vi "Set Excel Value.vi"(4 "Excel_Values":string[][](array[string]), 6 "SheetName(\"\")":string, 8 "error in (no error)":errorcluster, 9 "End":cluster{"Column":i32, "Row":i32}={"Column"=8, "Row"=7}, 10 "Start":cluster{"Column":i32, "Row":i32}={"Column"=1, "Row"=1}, 11 "path":path) -> (0 "error out":errorcluster)   [LabVIEW 2015]
uses:
  Private Methods/OpenXL_WorkSheet By Name.vi
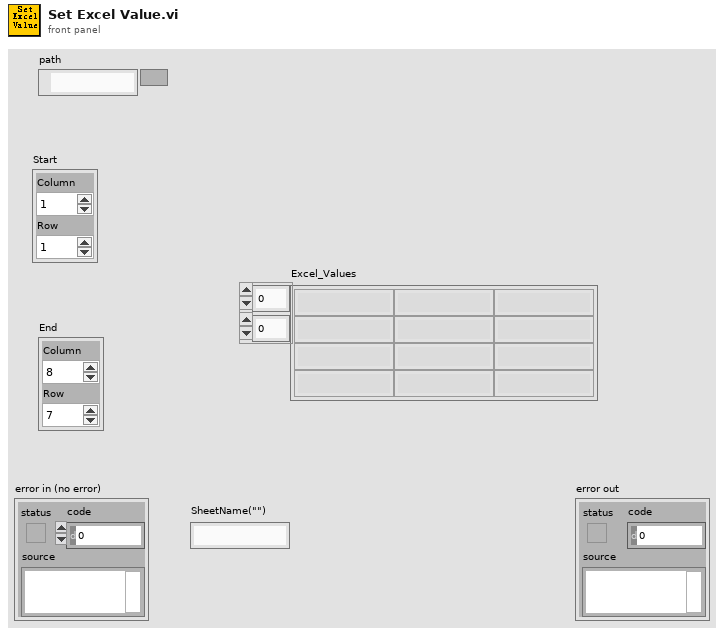
[diagram p1: front panel]
types:
  T1 = cluster{"Excel._Application":refnum<k7>, "Workbooks":refnum<k7>}
  T2 = cluster{"Excel._Application":refnum<k7>, "Workbooks":refnum<k7>, "Open":refnum<k7>}
  T3 = cluster{"Excel._Application":refnum<k7>, "Workbooks":refnum<k7>, "Open":refnum<k7>, "Worksheets":refnum<k7>, "Excel._Worksheet":refnum<k7>}
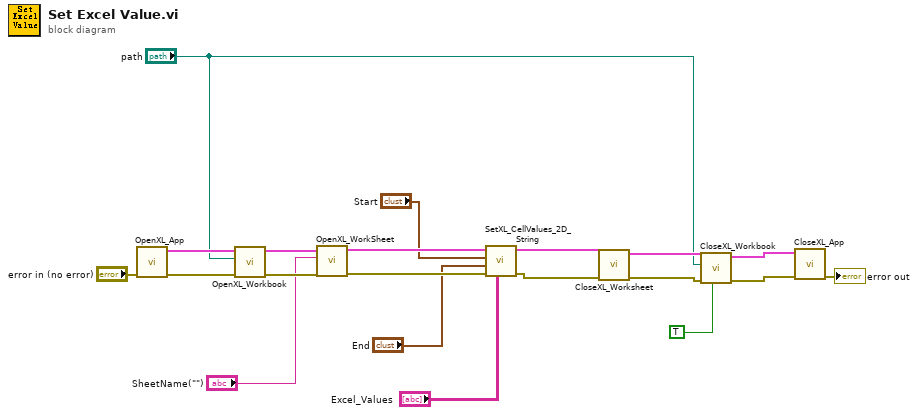
[diagram p0: block diagram]
diagram:
  n1 = call "OpenXL_App.vi"("error in (no error)"="error in (no error)") -> ("error out"=w19:errorcluster, "Refnum Cluster"=w20:T1)  [unwired: 9 in]
  n2 = call "OpenXL_Workbook.vi"("error in"=w19, "path"="path", "Refnum Cluster In"=w20) -> ("error out"=w11:errorcluster, "Refnum Cluster Out"=w12:T2)  [unwired: 7 in]
  n3 = call-poly "OpenXL_WorkSheet.vi"("error in (no error)"=w11, "SheetName(\"\")"="SheetName(\"\")", "Refnum Cluster In"=w12) -> ("error out"=w9:errorcluster, "Refnum Cluster Out"=w8:T3)  [unwired: 7 in]
  n4 = call "SetXL_CellValues_2D_String.vi"("data"="Excel_Values", "error in"=w9, "End"="End", "Start"="Start", "Refnum Cluster In"=w8) -> ("error out"=w6:errorcluster, "Refnum Cluster Out"=w7:T3)  [unwired: 5 in]
  n5 = call "CloseXL_Worksheet.vi"("error in (no error)"=w6, "Refnum Cluster In"=w7) -> ("error out"=w17:errorcluster, "Refnum Cluster Out"=w18:T2)  [unwired: 8 in]
  n6 = call "CloseXL_Workbook.vi"("Save? (F)"=TRUE, "error in (no error)"=w17, "path"="path", "Refnum Cluster In"=w18) -> ("error out"=w15:errorcluster, "Refnum Cluster Out"=w16:T1)  [unwired: 6 in]
  n7 = call "CloseXL_App.vi"("error in (no error)"=w15, "Refnum Cluster In"=w16) -> ("error out"=→"error out":errorcluster)  [unwired: 9 in]
